vi "createTopic.vi"(8 "error in (no error)":errorcluster, 9 "topicContentsString":string, 10 "topicName":string, 11 "Module in":refnum<class "Module.lvclass">) -> (0 "error out":errorcluster, 3 "Module out":refnum<class "Module.lvclass">)   [LabVIEW 2016, in "Module.lvclass"]
uses:
  Module.lvclass
  Topic/Topic.lvclass
  ElementFactory/ElementFactory/ElementFactory.lvclass
  D:/Code/ts_SALLabVIEW/SALTypeGenerator/ElementFactory/IElementFactory/IElementFactory.lvclass
  Topic/Topic.lvclass/Topic.ctl
  Module.lvclass/Module.ctl
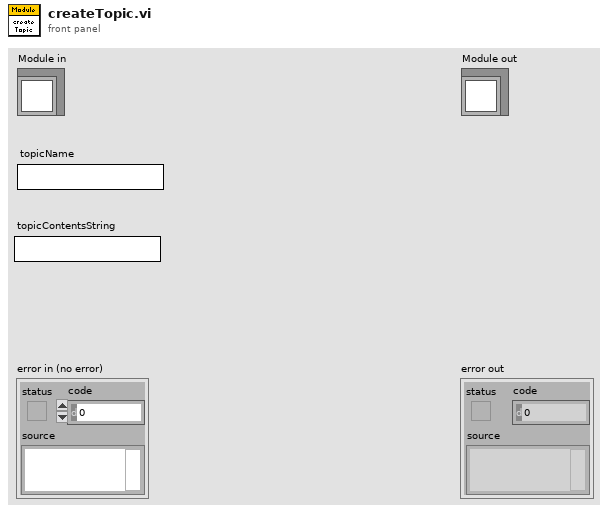
[diagram p1: front panel]
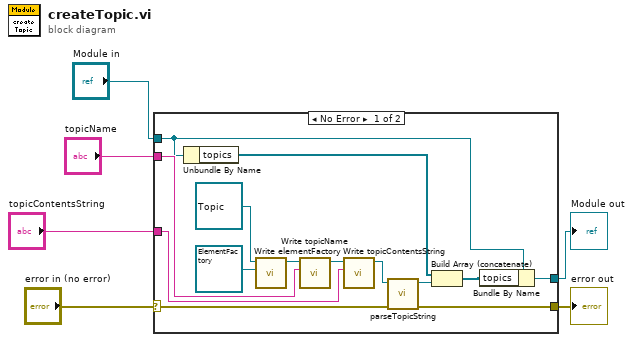
[diagram p0: block diagram]
diagram:
  n1 = case shown="No Error" "error in (no error)" {
    selector: "error in (no error)" -> [w14 w22]
    tunnel: [w13 w22] -> w5
    tunnel: [w10 w21] -> w3
    tunnel: "Module in" -> [w11 w21]
    tunnel: "topicName" -> [w16 _]
    tunnel: "topicContentsString" -> [w15 _]
    frame No Error {
      n2 = Unbundle By Name(w11) -> ("topics"=w9:refnum<class "Topic.lvclass">[])
      n3 = call "Write elementFactory.vi"("IElementFactory.lvclass"=refnum<class "ElementFactory.lvclass"> refnum ("ElementFactory.lvclass"), "Topic in"=refnum<class "Topic.lvclass"> refnum ("Topic.lvclass")) -> ("Topic out"=w19:refnum<class "Topic.lvclass">)  [unwired: 9 in]
      n4 = call "Write topicName.vi"("topicName"=w16, "Topic in"=w19) -> ("Topic out"=w17:refnum<class "Topic.lvclass">)  [unwired: 9 in]
      n5 = call "Write topicContentsString.vi"("topicContentsString"=w15, "Topic in"=w17) -> ("Topic out"=w12:refnum<class "Topic.lvclass">)  [unwired: 9 in]
      n6 = call "parseTopicString.vi"("error in (no error)"=w14, "Topic in"=w12) -> ("error out"=w13:errorcluster, "Topic out"=w8:refnum<class "Topic.lvclass">)  [unwired: 8 in]
      n7 = Build Array (concatenate)(w9, w8) -> (w7:refnum<class "Topic.lvclass">[])
      n8 = Bundle By Name(cluster=w11, "topics"=w7) -> (w10:refnum<class "Module.lvclass">)
    }
    frame Error {
    }
  }
  "error out" <- w5
  "Module out" <- w3
